vi "bluetoothTest.vi"() -> ()   [LabVIEW 2015]
uses:
  <vilib>/myRIO/Instrument Drivers/Onboard IO/UART/typedef/VISA Configuration.ctl
  <vilib>/Instr/_visa.llb/VISA Configure Serial Port (Instr).vi
  <vilib>/myRIO/Express VI/Onboard IO/UART/UART Express VI.xnode
  <vilib>/myRIO/Instrument Drivers/Onboard IO/UART/UART.lvlib
panel:
  out "match + rest of string":string
  out "Waveform Chart":i32(graph)
  out "Numeric":i32
  out "substring before match 2":string
  out "whole string":string
  in  "stop":bool
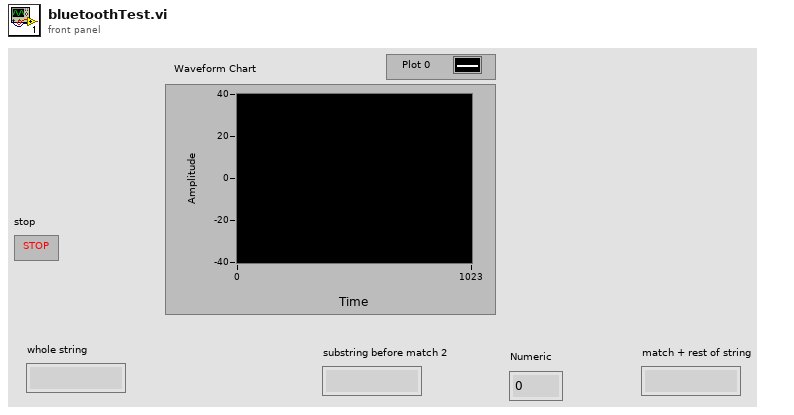
[diagram p1: front panel]
types:
  T1 = typedef "UART.lvlib/VISA Configuration.ctl" = cluster{"baud rate (9600)":u32, "data bits (8)":u16, "parity (0:none)":enum16{"None", "Odd", "Even", "Mark", "Space"}, "stop bits (10: 1 bit)":u16, "flow control (0:none)":u16, "termination char\n(0xA = '\\n' = LF) ":u8, "Enable Termination\nChar (T)":bool, "timeout (10sec)":u32}
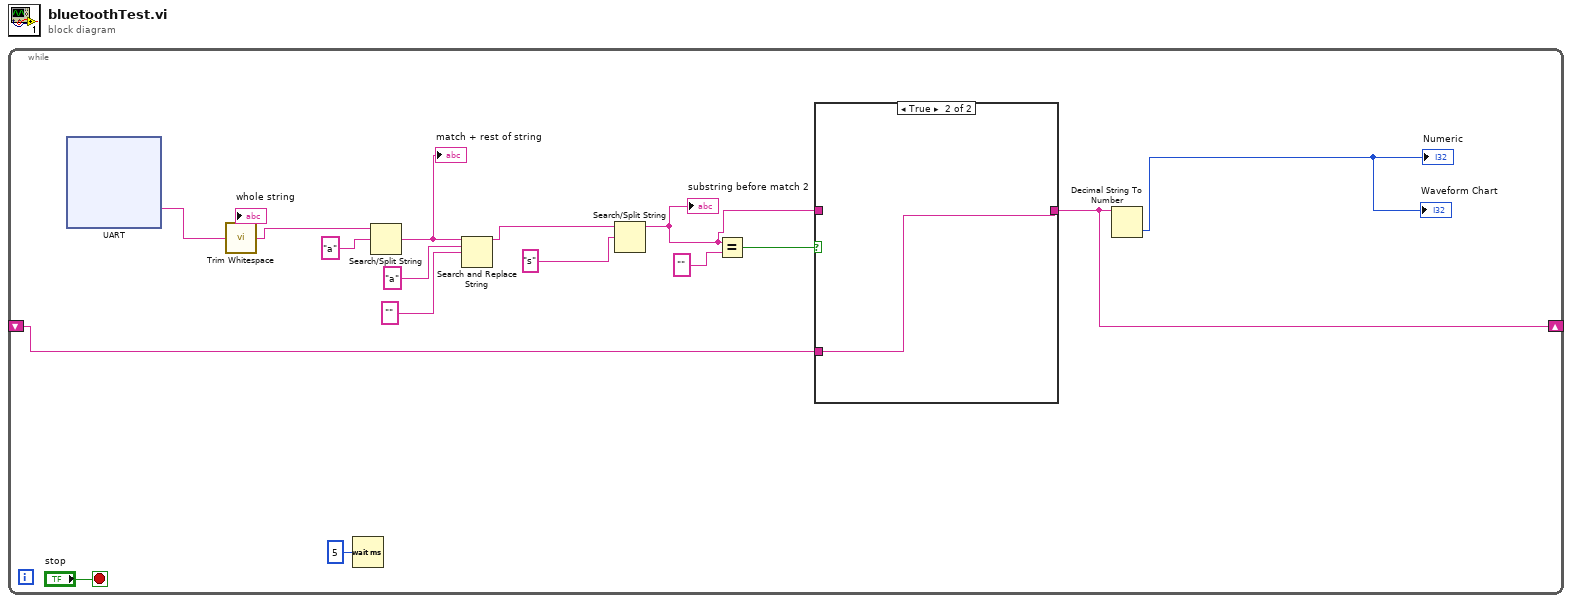
[diagram p0: block diagram]
diagram:
  n1 = while {
    shift-right: [w2] -> _
    shift-left: _ -> [w1]
    stop <- "stop" stop-if-true
    n2 = xnode "UART"() -> ("Characters Read"=w10:string)  [unwired: 1 in, 1 out]
    n3 = call <vilib>:"Trim Whitespace.vi"("string"=w10) -> ("trimmed string"=w9:string)  [unwired: 1 in]
    n4 = Wait (ms)(milliseconds to wait=u32 5) -> ()  [unwired: 1 out]
    n5 = Search/Split String(string=w9, search string/char (-)="a") -> (match + rest of string=w8:string)  [unwired: 1 in, 2 out]
    "match + rest of string" <- w8
    n6 = Search and Replace String(input string=w8, search string="a", replace string="" ("replace string (\"\")")) -> (result string=w7:string)  [unwired: 5 in, 3 out]
    n7 = Search/Split String(string=w7, search string/char (-)="s") -> (substring before match=w4:string)  [unwired: 1 in, 2 out]
    "substring before match 2" <- w4
    n8 = Equal?(x=w4, y="") -> (x = y?=w11:bool)
    n9 = case shown="True" w11 {
      tunnel: w4 -> [w17 _]
      tunnel: w1 -> [_ w18]
      tunnel: [w17 w18] -> w2
      frame False {
      }
      frame True {
      }
    }
    n10 = Decimal String To Number(string=w2) -> (number=→"Numeric" →"Waveform Chart":i32)  [unwired: 2 in, 1 out]
  }
